vi "GetDisplayName3.vi"(0 "XRef":T6, 1 "State In":T3) -> (14 "Type Name":T2, 15 "Instance Name":T2, 16 "Fatal Error Out":T1)   [LabVIEW 2021, in "FirstXNode .xnode"]
uses:
  FirstXNode .xnode
  <vilib>/XNodeSupport/XNodeXNodeRef.ctl
  State.ctl
  <vilib>/XNodeSupport/XNodeBounds.ctl
  <vilib>/XNodeSupport/XNodeInt.ctl
  <vilib>/XNodeSupport/XNodeString.ctl
  <vilib>/XNodeSupport/XNodeErrorCluster.ctl
  <vilib>/XNodeSupport/NI_XNodeSupport.lvlib
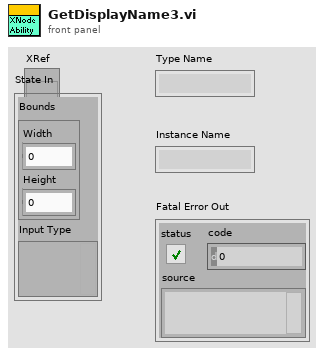
[diagram p1: front panel]
types:
  T1 = typedef "NI_XNodeSupport.lvlib/XNodeErrorCluster.ctl" = errorcluster
  T2 = typedef "NI_XNodeSupport.lvlib/XNodeString.ctl" = string
  T3 = typedef "FirstXNode .xnode/State.ctl" = cluster{"Bounds":T4, "Input Type":variant}
  T4 = typedef "NI_XNodeSupport.lvlib/XNodeBounds.ctl" = cluster{"Width":T5, "Height":T5}
  T5 = typedef "NI_XNodeSupport.lvlib/XNodeInt.ctl" = i32
  T6 = typedef "NI_XNodeSupport.lvlib/XNodeXNodeRef.ctl" = refnum<vi>
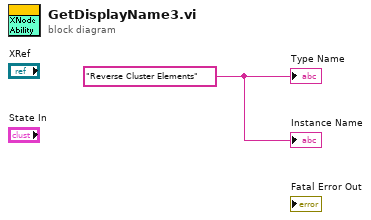
[diagram p0: block diagram]
diagram:
  w1 = T2 "Reverse Cluster Elements" ("Instance Name")
  "Type Name" <- w1
  "Instance Name" <- w1
